vi "Free.vi"(8 "error in (no error)":errorcluster, 11 "OpenSSL Context in":refnum<class "SSL Context.lvclass">) -> (0 "error out":errorcluster)   [LabVIEW 2013, in "OpenSSL Socket.lvlib" / "SSL Context.lvclass"]
uses:
  SSL Context.lvclass
  SSL Context.lvclass/SSL Context.ctl
  SSL_Lib/SSL-Context/SSL-Context.lvclass
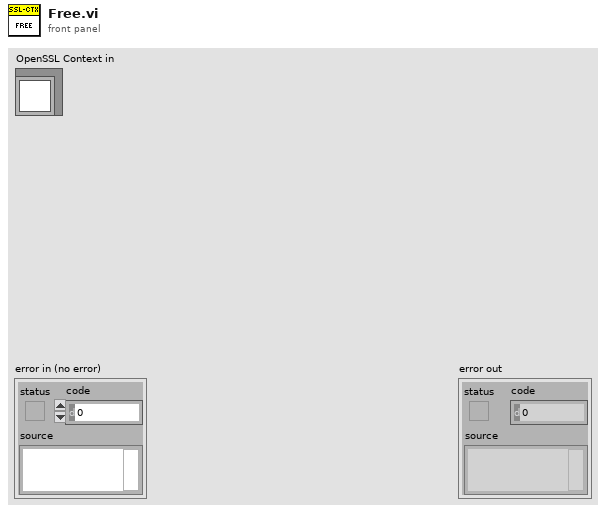
[diagram p1: front panel]
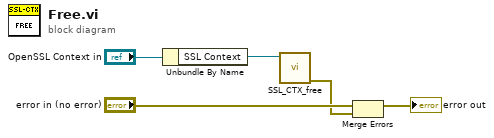
[diagram p0: block diagram]
diagram:
  n1 = Unbundle By Name("OpenSSL Context in") -> ("SSL Context"=w3:refnum<class "SSL-Context.lvclass">)
  n2 = call "SSL_CTX_free.vi"("SSL-Context in"=w3) -> ("error out"=w1:errorcluster)  [unwired: 10 in]
  n3 = Merge Errors("error in (no error)", w1) -> (→"error out":errorcluster)
